vi "GetLVFilesWithCompiledCode.vi"(6 "patterns":string[](array[string]), 8 "error in":errorcluster, 10 "Folders to Exclude":string[](array[string]), 11 "Search Path":path) -> (0 "error out":errorcluster, 3 "VIs with compiled code":path[](array[path]))   [LabVIEW 2017, in "VeriStandTestUtilities.lvlib"]
uses:
  VeriStandTestUtilities.lvlib
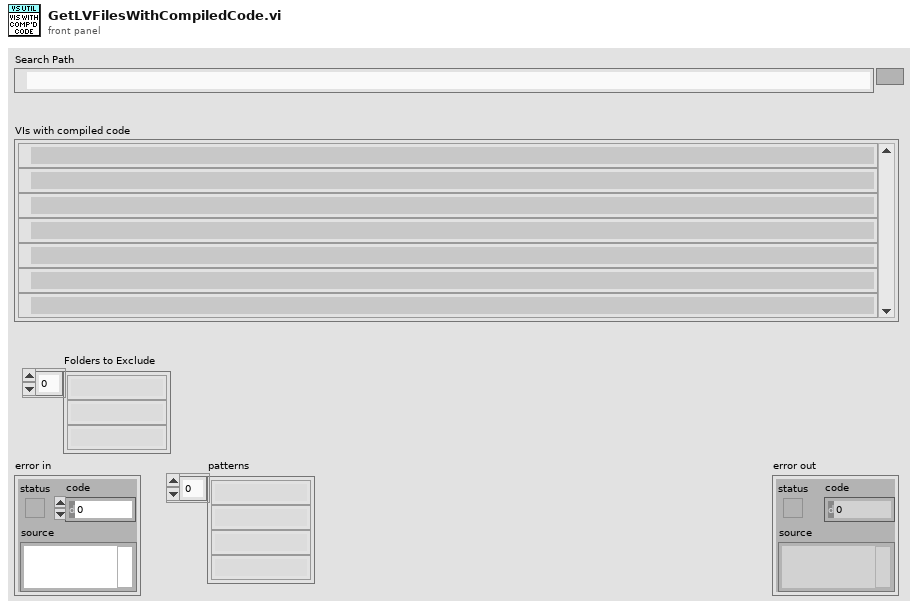
[diagram p1: front panel]
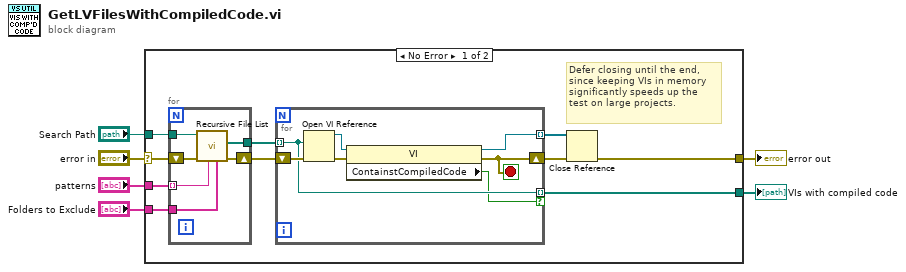
[diagram p0: block diagram]
diagram:
  n1 = case shown="No Error" "error in" {
    selector: "error in" -> [w13 w30]
    tunnel: [w8 w30] -> w6
    tunnel: "Search Path" -> [w15 _]
    tunnel: [w16 _] -> w3
    tunnel: "Folders to Exclude" -> [w11 _]
    tunnel: "patterns" -> [w7 _]
    frame No Error {
      # "Defer closing until the end,\nsince keeping VIs in memory\nsignificantly speeds up the\ntest on large projects."
      n2 = for {
        tunnel: w15 -> [w22]
        tunnel: [w21] -> w14
        tunnel: w11 -> [w18]
        shift-right: [w19] -> w12
        shift-left: w13 -> [w20]
        tunnel: w7 -> [w17] mode=indexing
        n3 = call <vilib>:"Recursive File List.vi"("Folders to Exclude"=w18, "pattern"=w17, "error in (no error)"=w20, "Folder Path"=w22) -> ("error out"=w19:errorcluster, "All Files in Dir"=w21:path[])  [unwired: 3 in, 3 out]
      }
      n4 = for {
        tunnel: w14 -> [w26] mode=indexing
        shift-right: [w24] -> w9
        shift-left: w12 -> [w29]
        tunnel: [w26] -> w16 mode=indexing if=w25
        tunnel: [w23] -> w10 mode=indexing
        stop <- w24 stop-if-true
        n5 = Open VI Reference(vi path=w26, error in (no error)=w29) -> (vi reference=w27:refnum<vi>, error out=w28:errorcluster)  [unwired: 4 in]
        n6 = property class="VI"(reference=w27, error in=w28) -> (reference out=w23:refnum<vi>, error out=w24:errorcluster, "ContainstCompiledCode"=w25:bool)
      }
      n7 = Close Reference(reference=w10, error in (no error)=w9) -> (error out=w8:errorcluster)
    }
    frame Error {
    }
  }
  "error out" <- w6
  "VIs with compiled code" <- w3
